vi "E4440A_PSA_Averaging.vi"(7 "Enable Averaging (T: Enable)":bool=TRUE, 8 "error in (no error)":errorcluster, 9 "Averaging Type (0: Auto)":u16(ring) items=["Auto", "RMS", "Video", "Scalar"], 10 "Average Count (100)":i32=100, 11 "VISA resource name":refnum<visa-resource-name>) -> (0 "error out":errorcluster, 3 "VISA resource name out":refnum<visa-resource-name>)   [LabVIEW 2015]
doc: "Configures the averaging."
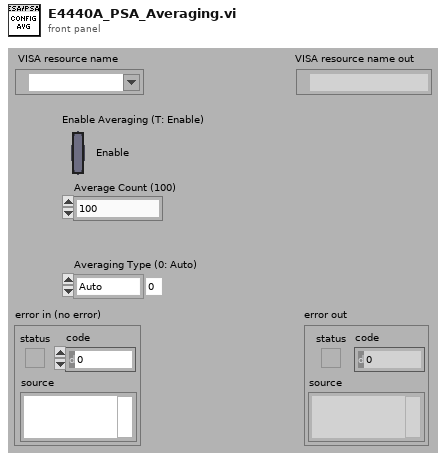
[diagram p1: front panel]
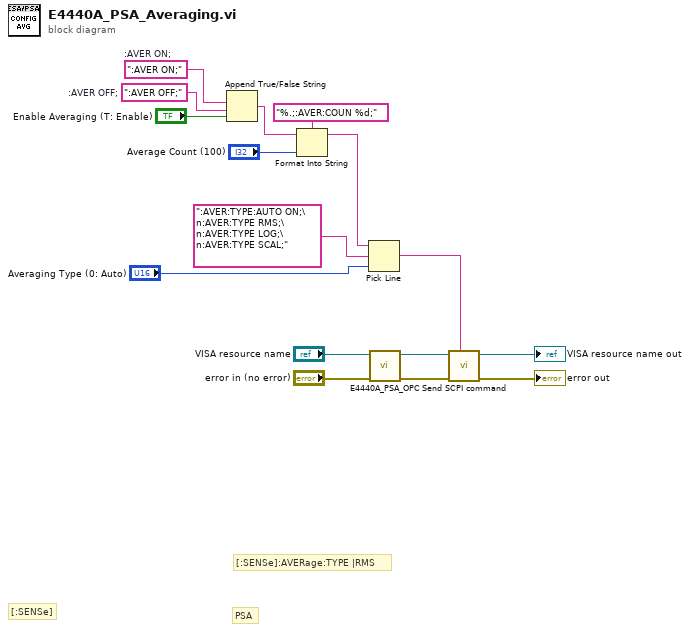
[diagram p0: block diagram]
diagram:
  w11 = ":AVER OFF;"  # :AVER OFF;
  w15 = ":AVER ON;"  # :AVER ON;
  # "PSA"
  # "[:SENSe]:AVERage:TYPE |RMS"
  # "[:SENSe]"
  n1 = Append True/False String(1:"Enable Averaging (T: Enable)", 2:w11, 3:w15) -> (0:w10:string)  [unwired: 1 in]
  n2 = Format Into String(format string="%.;:AVER:COUN %d;", initial string=w10, "Average Count (100)") -> (resulting string=w9:string)  [unwired: 1 in, 1 out]
  n3 = Pick Line(string ("")=w9, multi-line string=":AVER:TYPE:AUTO ON;\n:AVER:TYPE RMS;\n:AVER:TYPE LOG;\n:AVER:TYPE SCAL;", line index="Averaging Type (0: Auto)") -> (output string=w4:string)
  n4 = call "E4440A_PSA_OPC.vi"("error in (no error)"="error in (no error)", "VISA resource name"="VISA resource name") -> ("error out"=w3:errorcluster, "VISA resource name out"=w1:refnum<visa-resource-name>)  [unwired: 8 in]
  n5 = call "Send SCPI command.vi"("Send SCPI Command"=w4, "error in (no error)"=w3, "VISA resource name"=w1) -> ("error out"=→"error out":errorcluster, "VISA resource name out"=→"VISA resource name out":refnum<visa-resource-name>)  [unwired: 7 in]
